vi "Configure Digital Filter.vi"(0 "VISA resource name":refnum<visa-resource-name>, 1 "Enable Digital Filter (F: Disable)":bool caption="Enable Digital Filter", 5 "Filter Type (0: Moving)":i32(ring) items=["Moving", "Repeating"], 7 "Filter Count (10)":i32=10 min=2 max=320 step=1, 9 "Filter Window (2: 1%)":i32(ring)=2 items=["None", "10", "1", "0.1", "0.01"], 11 "error in (no error)":errorcluster) -> (4 "VISA resource name out":refnum<visa-resource-name>, 15 "error out":errorcluster)   [LabVIEW 2021, in "GWInstek  GDM8351.lvlib"]
doc: "Configures the type, count, window for digital filter."
uses:
  <instrlib>/GWInstek  GDM8351/GWInstek  GDM8351.lvlib
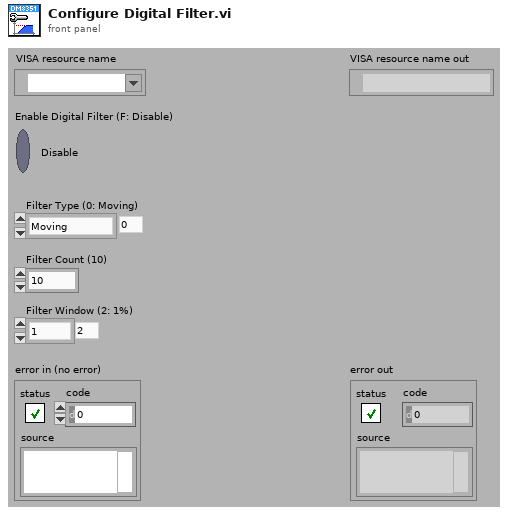
[diagram p1: front panel]
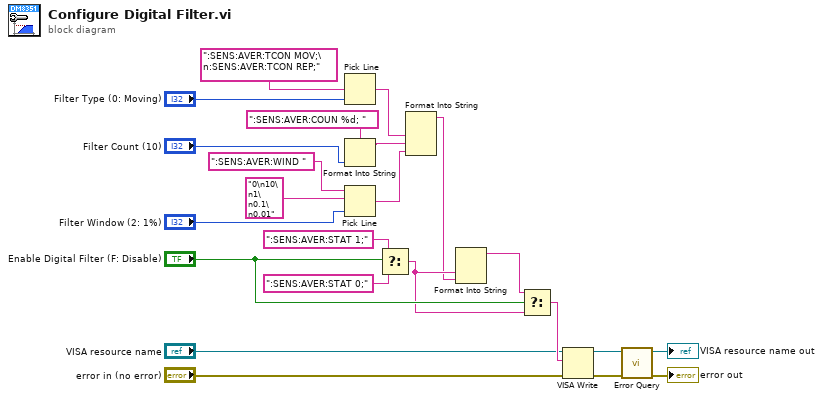
[diagram p0: block diagram]
diagram:
  n1 = Pick Line(multi-line string=":SENS:AVER:TCON MOV;\n:SENS:AVER:TCON REP;", line index="Filter Type (0: Moving)") -> (output string=w4:string)  [unwired: 1 in]
  n2 = Format Into String(format string=":SENS:AVER:COUN %d; ", "Filter Count (10)") -> (resulting string=w5:string)  [unwired: 2 in, 1 out]
  n3 = Pick Line(string ("")=":SENS:AVER:WIND ", multi-line string="0\n10\n1\n0.1\n0.01", line index="Filter Window (2: 1%)") -> (output string=w6:string)
  n4 = Select(t=":SENS:AVER:STAT 1;", s="Enable Digital Filter (F: Disable)", f=":SENS:AVER:STAT 0;") -> (s? t:f=w2:string)
  n5 = Format Into String(w4, w5, w6) -> (resulting string=w1:string)  [unwired: 3 in, 1 out]
  n6 = Format Into String(w2, w1) -> (resulting string=w3:string)  [unwired: 3 in, 1 out]
  n7 = Select(t=w3, s="Enable Digital Filter (F: Disable)", f=w2) -> (s? t:f=w13:string)
  n8 = VISA Write(VISA resource name="VISA resource name", write buffer=w13, error in (no error)="error in (no error)") -> (VISA resource name out=w10:refnum<visa-resource-name>, error out=w9:errorcluster)  [unwired: 1 out]
  n9 = call <instrlib>:"Error Query.vi"("error in (no error)"=w9, "VISA resource name"=w10) -> ("error out"=→"error out":errorcluster, "VISA resource name out"=→"VISA resource name out":refnum<visa-resource-name>)  [unwired: 6 in, 2 out]
